vi "Right Click Menu Configuration.vi"(7 "MCListbox Refnum":refnum<vi>, 8 "error in (no error)":errorcluster, 10 "Coords":T1, 11 "MenuRef":refnum<k9>) -> (0 "error out":errorcluster)   [LabVIEW 2016, in "Assert API Components.lvlib" / "Assert Display.lvlib" / "Main Display.lvlib" / "Main Display.lvclass"]
doc: "Called when the user does a right click on the multicolumn listbox - gets all the column headers from the configuration file and displays them in the right click menu"
uses:
  Main Display.lvclass
  <vilib>/Utility/miscctls.llb/LVPoint32TypeDef.ctl
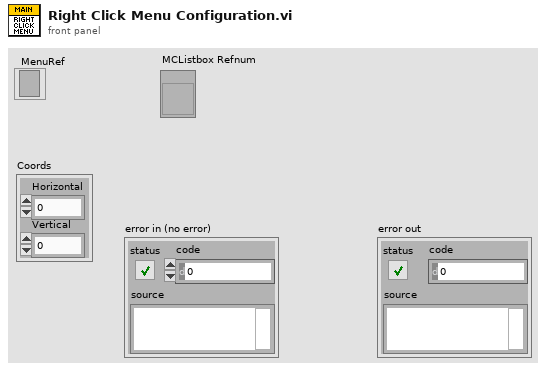
[diagram p1: front panel]
types:
  T1 = typedef "LVPoint32TypeDef.ctl" = cluster{"Horizontal":i32, "Vertical":i32}
  T2 = typedef "LVRowAndColumnTypeDef.ctl" = cluster{"Row":i32, "Column":i32}
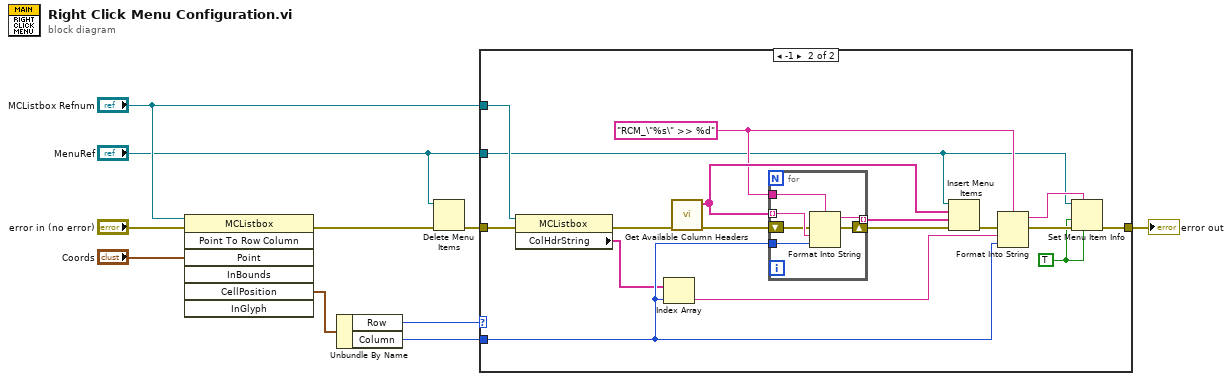
[diagram p0: block diagram]
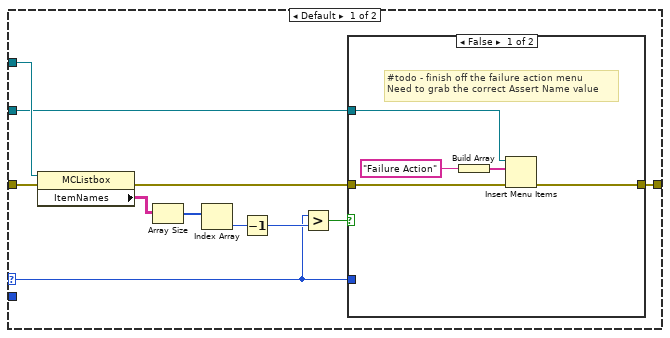
[diagram p2: hidden frame]
diagram:
  n1 = invoke on="Invoke Node" class="MCListbox" method="Point To Row Column"(reference="MCListbox Refnum", error in="error in (no error)", "Point"="Coords") -> (error out=w3:errorcluster, "CellPosition"=w8:T2)  [unwired: 4 in, 5 out]
  n2 = Unbundle By Name(w8) -> ("Row"=w6:i32, "Column"=w5:i32)
  n3 = Delete Menu Items(6:w3, 9:"MenuRef") -> (0:w7:errorcluster)  [unwired: 2 in, 1 out]
  n4 = case shown="-1" w6 {
    selector: w6 -> [w13 _]
    tunnel: [w11 w35] -> w9
    tunnel: "MenuRef" -> [w12 w28]
    tunnel: w7 -> [w21 w31]
    tunnel: w5 -> [_ w33]
    tunnel: "MCListbox Refnum" -> [w20 w32]
    frame Default {
      n5 = property class="MCListbox"(reference=w20, error in=w21) -> (error out=w14:errorcluster, "ItemNames"=w19:string[][])  [unwired: 1 out]
      n6 = Array Size(array=w19) -> (size(s)=w18:i32[])
      n7 = Index Array(array=w18) -> (element=w17:i32)  [unwired: 1 in]
      n8 = Decrement(x=w17) -> (x-1=w16:i32)
      n9 = Greater?(x=w13, y=w16) -> (0:w15:bool)
      n10 = case shown="False" w15 {
        tunnel: w14 -> [w26 w27]
        tunnel: w13 -> [_ _]
        tunnel: w12 -> [w24 _]
        tunnel: [w25 w27] -> w11
        frame False {
          # "#todo - finish off the failure action menu\nNeed to grab the correct Assert Name value"
          n11 = Build Array("Failure Action") -> (w22:string[])
          n12 = Insert Menu Items(6:w26, 8:w22, 9:w24) -> (0:w25:errorcluster)  [unwired: 3 in, 2 out]
        }
        frame True {
          # "Not clicked on an active assert row"
        }
      }
    }
    frame -1 {
      w34 = TRUE ("enabled")
      w39 = "RCM_\"%s\" >> %d" ("format string")
      n13 = property class="MCListbox"(reference=w32, error in=w31) -> (error out=w29:errorcluster, "ColHdrString"=w30:string[])  [unwired: 1 out]
      n14 = Index Array(array=w30, index=w33) -> (element=w38:string)
      n15 = call "Get Available Column Headers.vi"("error in (no error)"=w29) -> ("error out"=w42:errorcluster, "Available Column Headers"=w44:string[])  [unwired: 9 in]
      n16 = for {
        tunnel: w44 -> [w50] mode=indexing
        tunnel: [w49] -> w36 mode=indexing
        shift-right: [w47] -> w41
        shift-left: w42 -> [w48]
        tunnel: w39 -> [w46]
        tunnel: w33 -> [w45]
        n17 = Format Into String(format string=w46, error in=w48, w50, w45) -> (resulting string=w49:string, error out=w47:errorcluster)  [unwired: 1 in]
      }
      n18 = Insert Menu Items(6:w41, 7:w36, 8:w44, 9:w28) -> (0:w43:errorcluster)  [unwired: 2 in, 2 out]
      n19 = Format Into String(format string=w39, error in=w43, w38, w33) -> (resulting string=w37:string, error out=w40:errorcluster)  [unwired: 1 in]
      n20 = Set Menu Item Info(6:w34, 7:w37, 8:w40, 9:w34, 11:w28) -> (0:w35:errorcluster)  [unwired: 2 in, 1 out]
    }
  }
  "error out" <- w9
